vi "XYZWaveforms.vi"(3 "Colour Channel":dbl, 4 "Microscope Settings":T2={"Mode"=enum."X", "Slit"={"Scanning Mode"=0.0, "Slit Width /%"=0.0}, "Colour Channel"=enum."3", "Colour"=[], "Focus Offset /um"=0.0, "Exposure/ms"=0.0, "Piezo Position /um"=0.0, "ROI"={"X"={"Start /px"=0.0, "Step /px"=0.0, "Range /px"=0.0}, "Y"={"Start /px"=0.0, "Step /px"=0.0, "Range /px"=0.0}, "Z "={"Start /um"=0.0, "Step/um"=0.0, "Range /um"=0.0}, "T "={"Start /s"=0.0, "Step /s"=0.0, "Range /s"=0.0}}, "Samples per millisecond"=0.0, "Relax/ms"=0.0, "Readout Direction"=0.0, "Trigger Source"=0.0, "Camera Delay /ms"=0.0, "Under Scan /ms"=0.0, "Slit Delay"=100.0, "Waveforms"={"Analogue Out"=[], "Digital Out"=[]}} {"Focus Offset /um" min=0.0 max=10.0 step=0.05 scale=-2.0..2.0 scale format="%.2f"; "ROI"."T"."Range /s" min=0.0 max=10.0 step=0.05; "ROI"."T"."Step /s" min=0.0 max=10.0 step=0.05; "ROI"."T"."Start /s" min=0.0 max=10.0 step=0.05; "ROI"."X"."Range /px" min=0.0 max=10.0 step=0.05; "ROI"."X"."Step /px" min=0.0 max=10.0 step=0.05; "ROI"."X"."Start /px" min=0.0 max=10.0 step=0.05; "ROI"."Y"."Range /px" min=0.0 max=10.0 step=0.05; "ROI"."Y"."Step /px" min=0.0 max=10.0 step=0.05; "ROI"."Y"."Start /px" min=0.0 max=10.0 step=0.05; "ROI"."Z"."Range /um" min=0.0 max=10.0 step=0.05; "ROI"."Z"."Step/um" min=0.0 max=10.0 step=0.05; "ROI"."Z"."Start /um" min=0.0 max=10.0 step=0.05; "Colour"."Colour"."Filter" items=["Empty"=1, ""=2, ""=3, "561"=4, ""=5, "488"=6]; "Camera Delay /ms" min=0.0 max=10.0 step=0.05; "Trigger Source" items=["Internal"=1.0, "External"=2.0]; "Readout Direction" items=["Internal"=1.0, "External"=2.0]; "Slit"."Scanning Mode" items=["Full Frame"=1.0, "Slit Scanning"=12.0]; "Piezo Position /um" min=0.0 max=10.0 step=0.05; "Exposure/ms" min=0.0 max=10.0 step=0.05; "Samples per millisecond" min=1.0 max=2.0 step=1.0}) -> (0 "Analogue Out out":waveform(dbl)[](array[waveform]), 1 "Digital Out out":digitalwaveform[](array[waveform]))   [LabVIEW 2016]
uses:
  controls/Microscope Settings.ctl
  controls/ColourCalibration.ctl
  <vilib>/Waveform/DWDTOps.llb/DWDT Append Digital Samples.vi
  <vilib>/Waveform/WDTOps.llb/WDT Append Waveforms DBL.vi
panel:
  out "Mixed Signal Graph 2":waveform(dbl)(graph)
  out "dt":dbl
  out "Mixed Signal Graph":T1(graph)
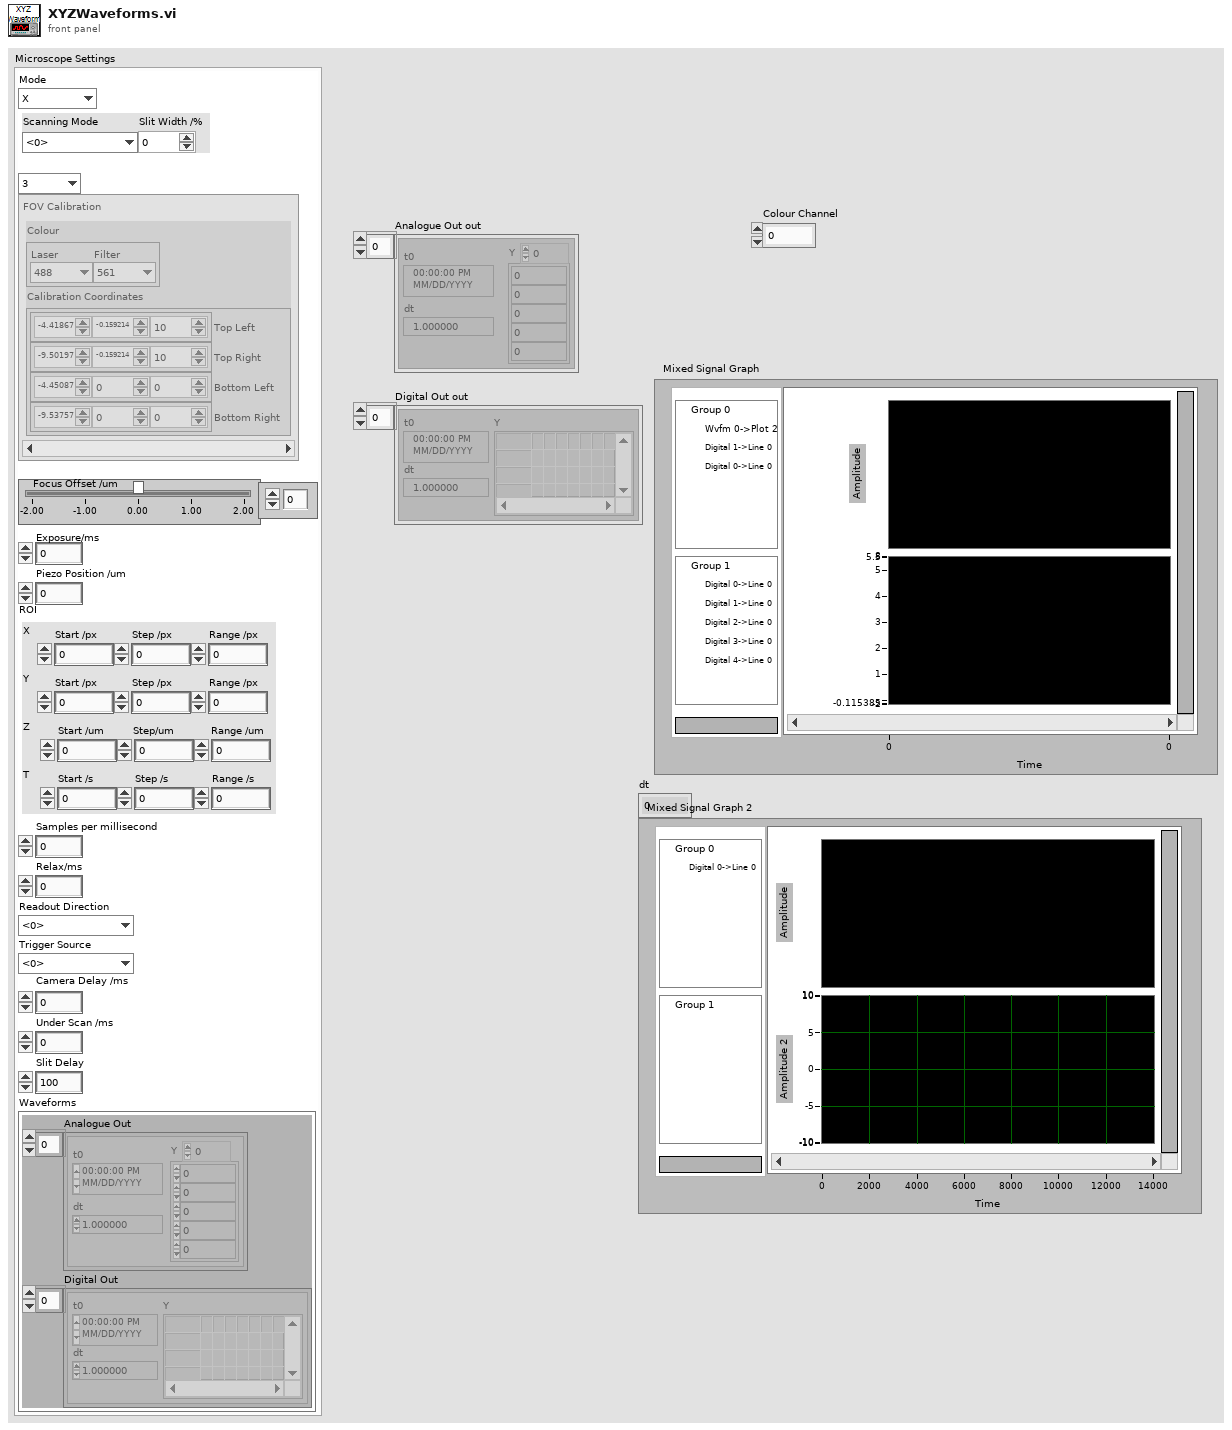
[diagram p1: front panel]
types:
  T1 = cluster{"Analogue Out":waveform(dbl)[], "Digital Out":digitalwaveform[]}
  T2 = typedef "Microscope Settings.ctl" = cluster{"Mode":enum16{"Brightfield", "X", "XY", "XYZ", "XYC", "XYCT", "XYZT", "XYZC", "Tweezers", "Virus"}, "Slit":cluster{"Scanning Mode":dbl, "Slit Width /%":dbl}, "Colour Channel":enum16{"1", "2", "3", "4", "5"}, "Colour":T3, "Focus Offset /um":dbl, "Exposure/ms":dbl, "Piezo Position /um":dbl, "ROI":cluster{"X":cluster{"Start /px":dbl, "Step /px":dbl, "Range /px":dbl}, "Y":cluster{"Start /px":dbl, "Step /px":dbl, "Range /px":dbl}, "Z ":cluster{"Start /um":dbl, "Step/um":dbl, "Range /um":dbl}, "T ":cluster{"Start /s":dbl, "Step /s":dbl, "Range /s":dbl}}, "Samples per millisecond":dbl, "Relax/ms":dbl, "Readout Direction":dbl, "Trigger Source":dbl, "Camera Delay /ms":dbl, "Under Scan /ms":dbl, "Slit Delay":dbl, "Waveforms":cluster{"Analogue Out":waveform(dbl)[], "Digital Out":digitalwaveform[]}}
  T3 = typedef "ColourCalibration.ctl" = cluster{"Colour":cluster{"Laser":enum16{"Brightfield", "445", "488", "561", "647"}, "Filter":u16}, "Calibration Coordinates":cluster{"Top Left":dbl[], "Top Right":dbl[], "Bottom Left":dbl[], "Bottom Right":dbl[]}}[]
  T4 = cluster{"Start /um":dbl, "Step/um":dbl, "Range /um":dbl}
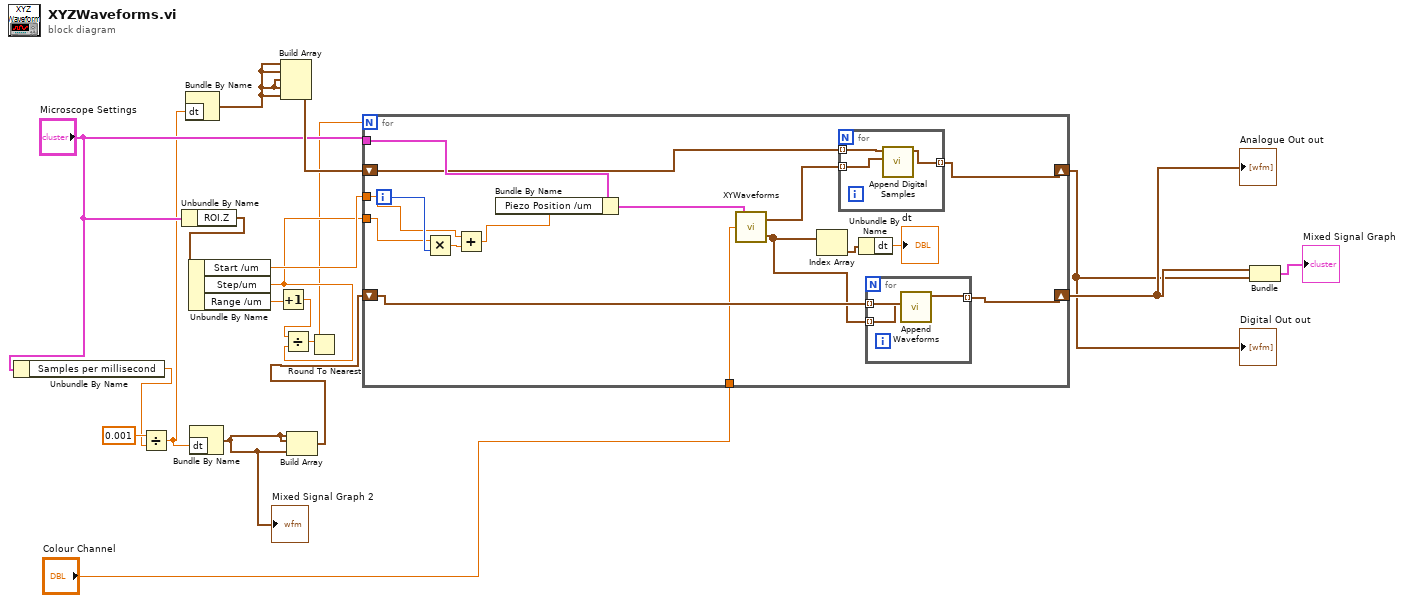
[diagram p0: block diagram]
diagram:
  n1 = Unbundle By Name("Microscope Settings") -> ("Samples per millisecond"=w8:dbl)
  n2 = Divide(x=0.001 ("y"), y=w8) -> (x/y=w6:dbl)
  n3 = Unbundle By Name("Microscope Settings") -> ("ROI.Z"=w19:T4)
  n4 = Bundle By Name("dt"=w6) -> (w5:digitalwaveform)  [unwired: 1 in]
  n5 = Unbundle By Name(w19) -> ("Start /um"=w18:dbl, "Step/um"=w17:dbl, "Range /um"=w2:dbl)
  n6 = Bundle By Name("dt"=w6) -> (w7:waveform(dbl))  [unwired: 1 in]
  "Mixed Signal Graph 2" <- w7
  n7 = Increment(x=w2) -> (x+1=w1:dbl)
  n8 = Build Array(w5, w5, w5, w5, w5) -> (w12:digitalwaveform[])
  n9 = Divide(x=w1, y=w17) -> (x/y=w16:dbl)
  n10 = Build Array(w7, w7, w7) -> (w11:waveform(dbl)[])
  n11 = Round To Nearest(number=w16) -> (nearest integer value=w3:dbl)
  n12 = for {
    N: w3 -> [_]
    tunnel: "Microscope Settings" -> [w35]
    tunnel: w17 -> [w31]
    tunnel: w18 -> [w30]
    shift-right: [w27] -> w15
    shift-left: w11 -> [w28]
    shift-right: [w25] -> w13
    shift-left: w12 -> [w24]
    tunnel: "Colour Channel" -> [w20]
    i -> [w32]
    n13 = Multiply(x=w31, y=w32) -> (x*y=w33:dbl)
    n14 = Add(x=w30, y=w33) -> (x+y=w29:dbl)
    n15 = Bundle By Name(cluster=w35, "Piezo Position /um"=w29) -> (w34:T2)
    n16 = call "XYWaveforms.vi"("Colour Channel"=w20, "Microscope Settings"=w34) -> ("Analogue Out"=w23:waveform(dbl)[], "Digital Out"=w26:digitalwaveform[])  [unwired: 1 out]
    n17 = Index Array(array=w23) -> (element=w22:waveform(dbl))  [unwired: 1 in]
    n18 = for {
      tunnel: w26 -> [w37] mode=indexing
      tunnel: w24 -> [w38] mode=indexing
      tunnel: [w36] -> w25 mode=indexing
      n19 = call-poly <vilib>:"Append Digital Samples.vi"("digital waveform B"=w37, "digital waveform A"=w38) -> ("digital waveform out"=w36:digitalwaveform)  [unwired: 8 in, 1 out]
    }
    n20 = Unbundle By Name(w22) -> ("dt"=→"dt":dbl)
    n21 = for {
      tunnel: w23 -> [w40] mode=indexing
      tunnel: w28 -> [w41] mode=indexing
      tunnel: [w39] -> w27 mode=indexing
      n22 = call-poly <vilib>:"Append Waveforms.vi"("waveform B"=w40, "waveform A"=w41) -> ("waveform out"=w39:waveform(dbl))  [unwired: 8 in, 1 out]
    }
  }
  "Analogue Out out" <- w15
  "Digital Out out" <- w13
  n23 = Bundle(w15, w13) -> (→"Mixed Signal Graph":cluster{waveform(dbl)[], digitalwaveform[]})  [unwired: 1 in]
